vi "PH_HamamatsuCamera.evt call Cam Parameter Write.vi"(0 "i ref in":refnum<vi>, 1 "Instance":string, 2 "Parameter to set":string, 3 "Value":dbl, 5 "error in (no error)":errorcluster) -> (14 "i ref out":refnum<vi>, 19 "error out":errorcluster)   [LabVIEW 2014, in "PH_HamamatsuCamera.lvlib"]
doc: "This VI sends a simple call for writing a camera attribute."
uses:
  PH_HamamatsuCamera.lvlib
  CS_Core/CSSystem/CoreLib/CoreLib.double 2 byte array.vi
  CS_Core/CSSystem/CoreLib/CoreLib.string 2 byte array.vi
  CS_Core/CSSystem/CoreLib/CoreLib.lvlib
  CS_Core/BaseProcess/BaseProcess.lvlib
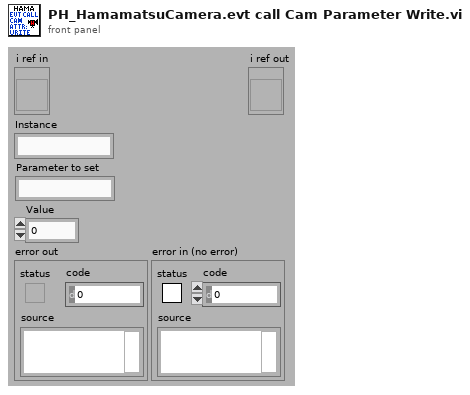
[diagram p1: front panel]
types:
  T1 = typedef "CoreDefs.rawDataType.ctl" = i8[]
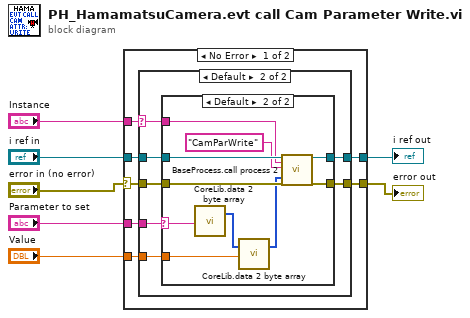
[diagram p0: block diagram]
diagram:
  n1 = case shown="No Error" "error in (no error)" {
    selector: "error in (no error)" -> [w11 w36]
    tunnel: [w14 w37] -> w4
    tunnel: [w13 w36] -> w3
    tunnel: "i ref in" -> [w12 w37]
    tunnel: "Instance" -> [w10 _]
    tunnel: "Value" -> [w9 _]
    tunnel: "Parameter to set" -> [w8 _]
    frame No Error {
      n2 = case shown="Default" w10 {
        selector: w10 -> [_ w18]
        tunnel: [w16 w23] -> w14
        tunnel: [w15 w22] -> w13
        tunnel: w12 -> [w16 w21]
        tunnel: w11 -> [w15 w20]
        tunnel: w9 -> [_ w19]
        tunnel: w8 -> [_ w17]
        frame "N/A" {
        }
        frame Default {
          n3 = case shown="Default" w17 {
            selector: w17 -> [_ w26]
            tunnel: [w25 w35] -> w23
            tunnel: [w24 w34] -> w22
            tunnel: w21 -> [w25 w33]
            tunnel: w20 -> [w24 w31]
            tunnel: w19 -> [_ w30]
            tunnel: w18 -> [_ w28]
            frame "", "N/A" {
            }
            frame Default {
              n4 = call-poly "CoreLib.data 2 byte array.vi"("string"=w26) -> ("byteArray out"=w29:T1)  [unwired: 18 in]
              n5 = call-poly "CoreLib.data 2 byte array.vi"("byteArray"=w29, "f64"=w30) -> ("byteArray out"=w27:T1)  [unwired: 17 in]
              n6 = call "BaseProcess.call process 2.vi"("i ref in"=w33, "Object"=w28, "Selector"="CamParWrite", "Data"=w27, "error in (no error)"=w31) -> ("i ref out"=w35:refnum<vi>, "error out"=w34:errorcluster)  [unwired: 13 in]
            }
          }
        }
      }
    }
    frame Error {
    }
  }
  "error out" <- w3
  "i ref out" <- w4
